vi "Dashboard Main.vi"() -> ()   [LabVIEW 2019]
uses:
  <vilib>/Rock Robotics/WPI/Camera/WPI_CameraSettings Read MJPG.ctl
  <vilib>/Rock Robotics/WPI/Camera/WPI_CameraImageSize.ctl
  Support Code/Adaptive Diagnostics/AD Status.ctl
  <vilib>/Rock Robotics/Network Tables/NT Read Number.vi
  <vilib>/Rock Robotics/Network Tables/NT Read Variant.vi
  <vilib>/Rock Robotics/Network Tables/NT Read Boolean.vi
  <vilib>/Rock Robotics/WPI/Dashboard/WPI_DashboardLogging Global.vi
  <vilib>/picture/picture.llb/Draw True-Color Pixmap.vi
  <vilib>/Rock Robotics/Network Tables/NT Read String Array.vi
  <vilib>/Rock Robotics/Network Tables/NT Write String Array.vi
  <vilib>/Rock Robotics/Network Tables/NT Write Boolean.vi
  <vilib>/Utility/miscctls.llb/LVPointTypeDef.ctl
  <vilib>/Utility/miscctls.llb/LVBoundsTypeDef.ctl
  <vilib>/FTP/NI_FTP.lvlib
  <vilib>/Rock Robotics/Network Tables/NT Write Number.vi
  <vilib>/Rock Robotics/Network Tables/NT Read String.vi
panel:
  in  "Enum":T1
  out "Camera Perf":string
  out "Right Camera Perf":cluster{"Bandwidth (Mbps)":dbl, "FPS":dbl}
  in  "Camera Settings Right":T2={"Frame Rate"=30, "Compression"=30, "Size"=1, "DB Camera Config"=FALSE} {"Frame Rate" scale=1.0..30.0; "Compression" scale=100.0..-1.0; "Size" items=["640x480", "320x240", "160x120"]}
  in  "Camera Name Right":string(combo)="No Camera Selection"
  in  "TCP":refnum<k5>
  in  "Rec Mode":enum32{"Stop", "Record", "Playback"}(radio)
  out "Robot IP":string
  in  "Dashboard Tab":T3(tab)
  out "NT 1":bool
  out "IMU 1":bool
  out "AD 1":bool
  out "Target Angle":dbl
  out "Actual Angle":dbl
  out "Target RPM":dbl
  out "Actual RPM":dbl
  in  "Camera Settings":T4={"fps"=30, "compression"=30, "Image Size"=enum."320x240", "Config Shown"=FALSE}
  out "Time Remaining":dbl
  out "Camera Image Right":T6(plugin-control)
  out "Endgame?":bool
  in  "Starting Position":bool
  in  "Remove Item":bool
  in  "Selected Item":i64
  in  "Name":string
  in  "Save":bool
  in  "Preset Auto":u16(ring) items=["3 and 3 - Left - U - Border"=1, "3 and 3 on the run- Left - U - Border"=2, "6 Ball - Center - S - Trench"=3, "6 Ball - Left - U - Border"=4, "8 Ball - Left Trench"=5, "8 Ball Right-Side"=6, "Auto test"=7, "Circles for Days"=8, "Newest"=9, "Test Code"=10, "test new"=11]
  in  "Auto Selection":u16[](array[ring]) items=["(0) 10 ft {5v 10a 0s 0f}"=1, "(0) Circle thing EXP"=2, "(0) Circle thing End"=3, "(0) Circle thing Middle"=4, "(0) Circle thing Start"=5, "(0) Circle thing {4v 20a 0s 0f}"=6, "(1) Off of hab {5v 10a 0s 5f}"=7, "0000 - REMOVE - 0000"=8, "10 feet"=9, "2056 Style Hatch Movement"=10, "Auto test 2"=11, "Auto-Builder-Test"=12, "Backup (V2) {6v, 15a, 0s. 0f}"=13, "Backup (V3) {6v, 15a, 0s. 0f}"=14, "Backup {6v, 15a, 0s. 0f}"=15, "C to shoot - Left Trench to Left Border"=16, "C to shoot - Left border"=17, "C to shoot - Trenchside border"=18, "Cargo Movement 1"=19, "Cargo Movement 2"=20, "Move to Back Trench - Front Trench"=21, "Move to Front Trench - Back Trench"=22, "Move to Front Trench for Center Port - Back Trench"=23, "Move to Front Trench for Center Port For 8 ball - Back Trench"=24, "Move to pick up 3 - Left border"=25, "Only pick up 3 - Left border"=26, "Pick up 2 - Left Trench"=27, "Pick up 2- Trenchside border"=28, "Pick up 3 - Left border"=29, "Pick up 3 - On the run border"=30, "Pick up 3 - Trench"=31, "Pick up 3 - Trench J"=32, "Pick up 3 - Trench S"=33, "Pick up 3 - Trench S + 2"=34, "Pick up 3 - Trench S + C"=35, "Pick up 3 - Trench S for 8 Ball Auto"=36, "Pick up 3 test"=37, "Shoot 3 - Center Init Line"=38, "Shoot 3 - Center Init Line Facing Left"=39, "Shoot 3 - Center Init Line Strait"=40, "Shoot 3 - Front Trench"=41, "Shoot 3 - Front and side of trench"=42, "Shoot 3 - Front and side of trench and pickup"=43, "Shoot 3 - Side of Trench"=44, "Shoot 3 and 3 - Center Init Line Facing Left"=45, "Shoot 3 and 3 - Center Init Line Facing Right"=46, "Shoot 3 and 3 on the run - Center Init Line Facing Left"=47, "Test part 1"=48, "Test part 2"=49, "Turn in place and shoot"=50, "Untitled"=51]
  in  "Re-Calibrate":bool
  out "IMU Temp":dbl
  out "Gauge":dbl(knob) scale=-10.0..10.0
  out "Picture 2":picture
  out "Mode":T7(ring)=enum."Auto Disabled"
  out "IMU Angle":dbl
  out "Network Table 2":bool
  out "IMU 2":bool
  out "Adaptive Diagnostics 2":bool
  out "Drive Base":bool
  out "Turret":bool
  out "Shooter":bool
  out "Accelerator":bool
  out "Transfer":bool
  out "Funnel":bool
  out "Intake Rotation":bool
  out "Intake Power":bool
  out "Hang":bool
  out "Clang":bool
  out "Errors":string
  out "Front Left US":bool
  out "Back Left US":bool
  out "Front Right US":bool
  out "Back Right US":bool
  out "Beam-break":bool
  out "Limellight":bool
  out "Basler":bool
  in  "AD Save Path":path
  out "Network Table 3":bool
  out "IMU 3":bool
  out "Adaptive Diagnostics 3":bool
  out "Tree":string(tree)
  # "Straight on"
  # "Jail for random constants and stuff"
  # "HW"
  # "Preset Auto Selection"
  # "Robot Health"
  # "These only run when in the programming tab"
  # "Motors show if they detect non-\nzero encoder velocity"
  # "<Side pic of robot>"
  # "US shows <10"
  # "BB shows break"
  # "LL shows coms"
  # "<Top pic of robot>"
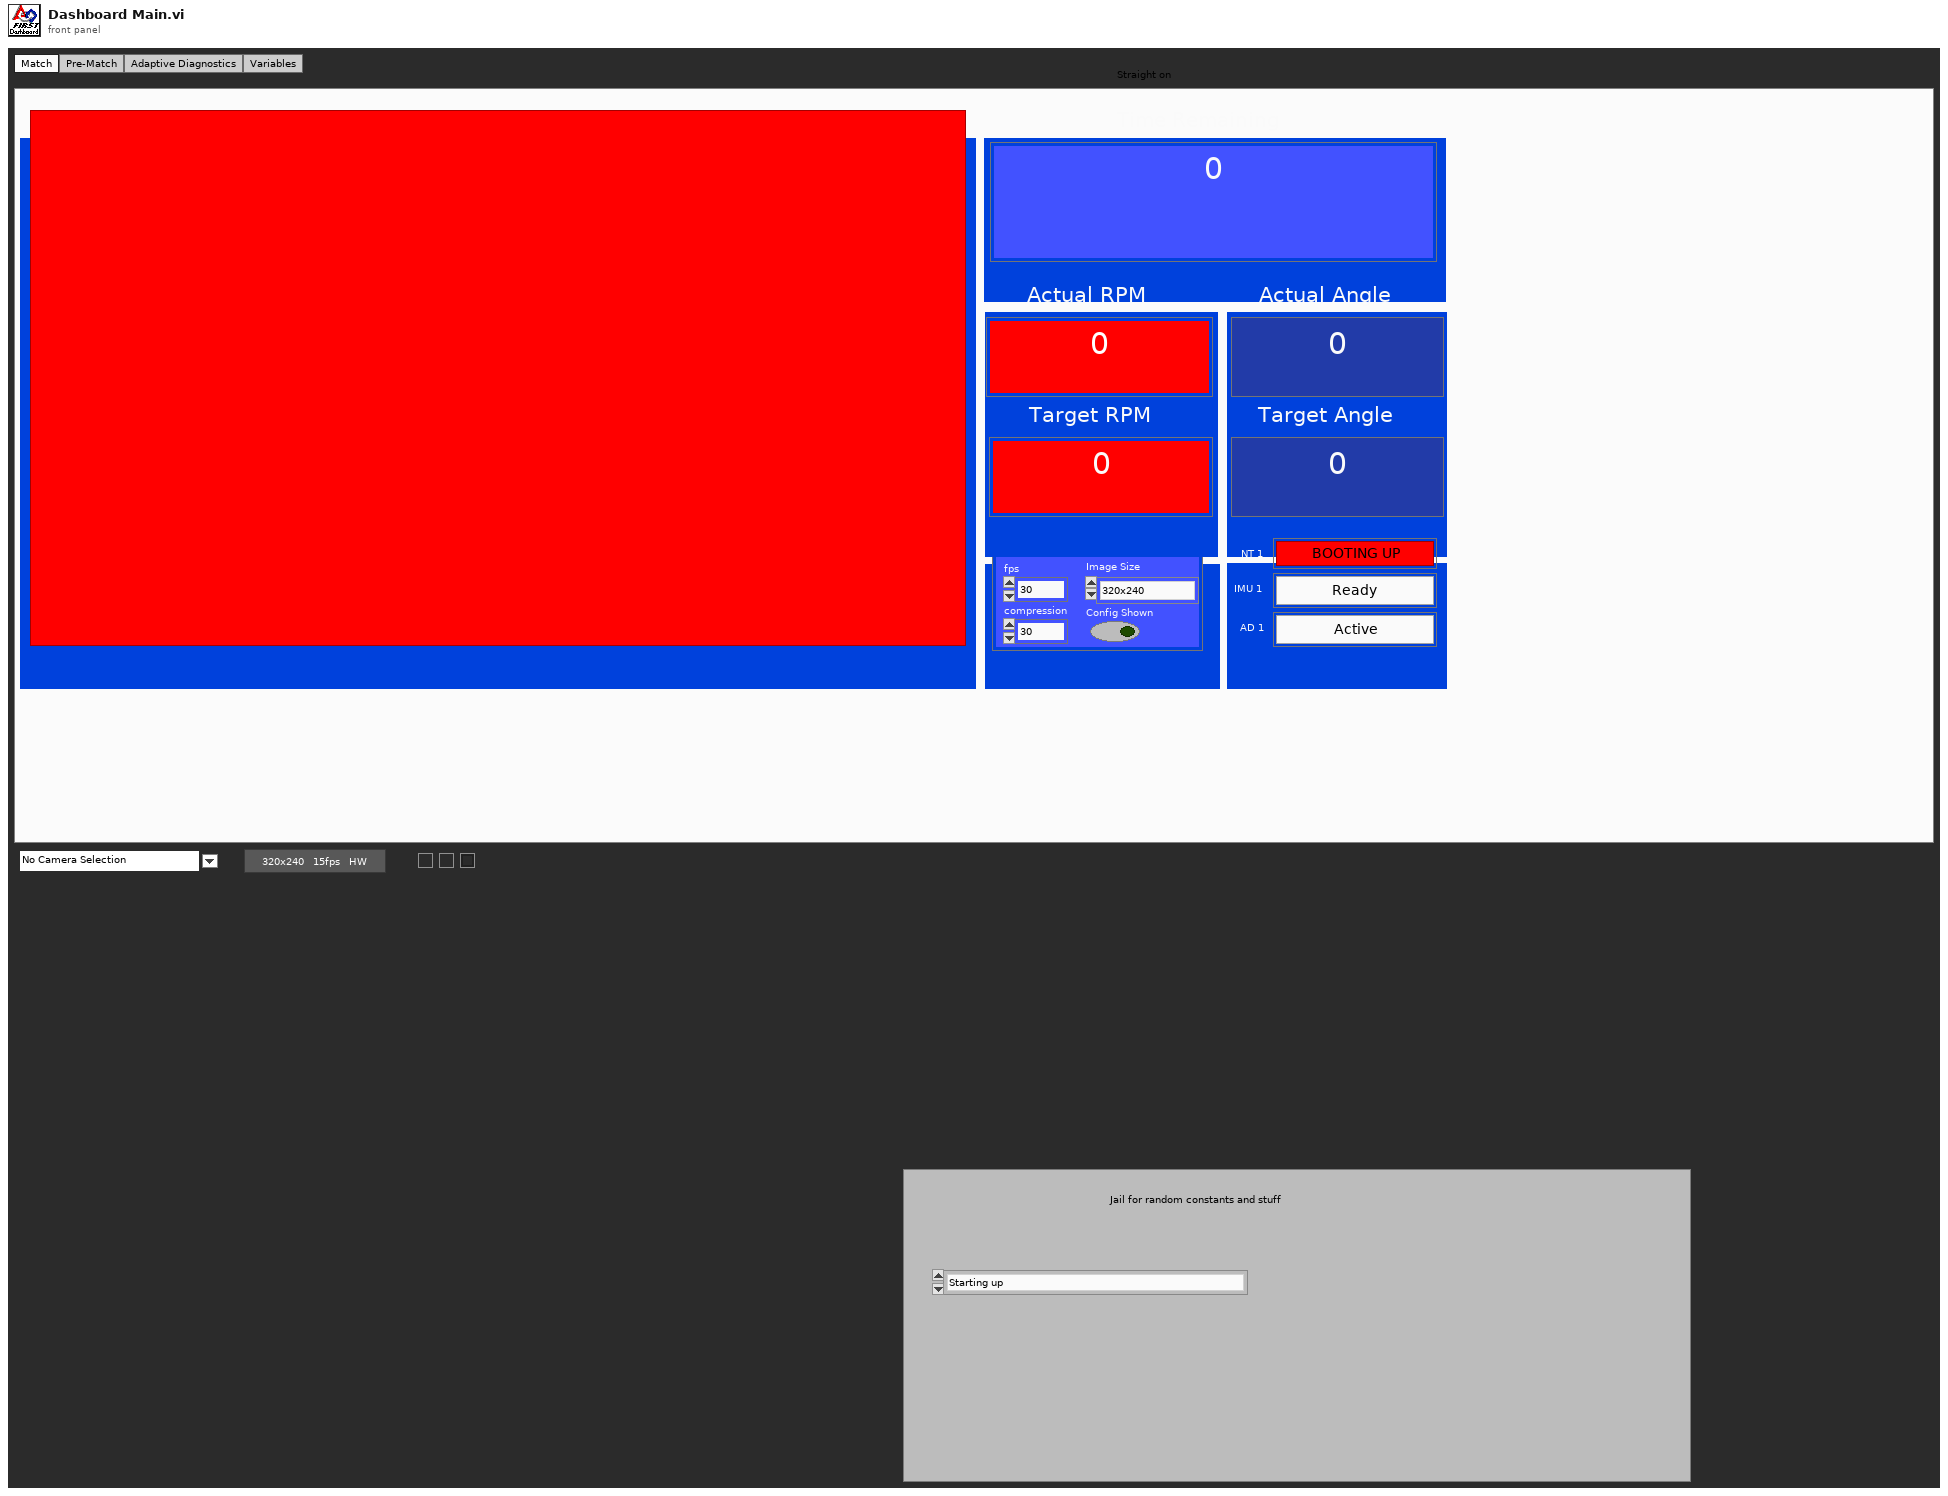
[diagram p1: front panel]
types:
  T1 = typedef "AD Status.ctl" = enum16{"Starting up", "Active", "Transfering Data", "Done"}
  T2 = cluster{"Frame Rate":i32, "Compression":i32, "Size":u16, "DB Camera Config":bool}
  T3 = enum32{"Match", "Pre-Match", "Adaptive Diagnostics", "Variables"}
  T4 = typedef "WPI_CameraSettings Read MJPG.ctl" = cluster{"fps":i32, "compression":i32, "Image Size":T5, "Config Shown":bool}
  T5 = typedef "WPI_CameraImageSize.ctl" = enum16{"640x480", "320x240", "160x120", "Custom"}
  T6 = typedef "IMAQ Image.ctl" = refnum<image>
  T7 = enum8{"Tele-Op Disabled", "Tele-Op Enabled", "Auto Disabled", "Auto Enabled", "Test Disabled", "Test Enabled", "Disconnected", "No Code", "E-Stop"}
  T8 = cluster{"Save Path":path, "Interval (s)":dbl, "Keep":i32}
  T9 = typedef "Image Type" = u32
  T10 = cluster{"IDs":cluster{"RPC field ID":u16, "Unique ID":u16}, "String":string}
  T11 = enum32{"Drive", "Camera", "Basic", "Custom", "Test", "Commands", "Checklist", "Variables"}
  T12 = cluster{"Segment Name":string, "Type":enum16{"Accel Straight", "Const Straight", "Blend", "Circle"}, "Traj Pos Points":cluster{"x":dbl, "y":dbl, "th":dbl}[], "Traj Vel Points":cluster{"V":dbl, "th":dbl}[], "Accel Index":i32, "Decel Index":i32}[]
  T13 = cluster{"Index":i32, "Pt Test Results":enum16{"Miss", "Rect Hit", "Arrow Hit"}}
  T14 = cluster{"Error Strings":string, "Disable Counts":cluster{u16, u16}, "Rail Faults":cluster{u16, u16, u16}, "Robot IP":string, "DB Mode":u8, "Event Info":cluster{"Name":string, "Type":u8, "Number":u16, "Replay":u8}}
  T15 = cluster{"Storage":cluster{"Disk Free":u64, "RAM Block":u32, "RAM free":u32}, "CPU Utilization":cluster{"CPU % ISR":sgl, "CPU % Time Crit":sgl, "CPU % Timed Str":sgl, "CPU % High":sgl, "CPU % Above":sgl, "CPU % Normal":sgl, "CPU % Low":sgl}, "CAN":cluster{"% Bus Utilization":sgl, "Bus Off Cnt":u32, "TX_FIFO Full Cnt":u32, "Receive Error Cnt":u8, "Transmit Error Cnt":u8}, "HID":cluster{"HID Outputs":u32, "Rumble Low":u16, "Rumble High":u16}[]}
  T16 = cluster{"Status bits":cluster{"Test Mode":bool, "Autonomous":bool, "Enabled":bool, "Code Start":bool, "Brownout":bool, "Reserved 2":bool, "Reserved 3":bool, "E-Stop":bool}, "Code Trace":cluster{"Disabled":bool, "TeleOp":bool, "Auto":bool, "Test":bool}, "Controller Type":enum16{"unknown", "cRIO", "roboRio"}, "Code?":enum16{"unknown", "noCode", "code"}, "Battery V":dbl}
  T17 = cluster{"Control Bits":cluster{"TestMode":bool, "Autonomous":bool, "Enabled":bool, "FMS Present":bool, bool, bool, bool, "E-Stop":bool}, "Team Station ":u8, "Countdown":sgl, "Joystick Values":cluster{"Axes":dbl[], "Buttons":bool[], "POVs":i16[]}[]}
  T18 = cluster{"Axes":dbl[], "Buttons":bool[], "POVs":i16[]}[]
  T19 = cluster{"Points":cluster{"x":dbl, "y":dbl, "th":dbl}[], "Trajectory Data":cluster{"Segment Name":string, "Type":enum16{"Accel Straight", "Const Straight", "Blend", "Circle"}, "Traj Pos Points":cluster{"x":dbl, "y":dbl, "th":dbl}[], "Traj Vel Points":cluster{"V":dbl, "th":dbl}[], "Accel Index":i32, "Decel Index":i32}[]}
  T20 = cluster{"Points":cluster{"x":dbl, "y":dbl, "th":dbl}[], "Trajectory Data":cluster{"Segment Name":string, "Type":enum16{"Accel Straight", "Const Straight", "Blend", "Circle"}, "Traj Pos Points":cluster{"x":dbl, "y":dbl, "th":dbl}[], "Traj Vel Points":cluster{"V":dbl, "th":dbl}[], "Accel Index":i32, "Decel Index":i32}[]}[]
  T21 = cluster{"Horizontal":dbl, "Vertical":dbl, "th":dbl}
  T22 = cluster{"Axes":dbl[], "Buttons":bool[], "POVs":i16[]}
  T23 = cluster{"Global Rectangle":i32[], "Contours":cluster{"Contour Type":u32, "ROI Type":u32, "Points":i32[]}[]}
  T24 = cluster{"Camera Name Right":string, string, "Saved DB Images Info":cluster{"Save Path":path, "Interval (s)":dbl, "Keep":i32}}
  T25 = cluster{"Operation":enum16{"Update", "Clear"}, "Color Box":u32}[]
  T26 = cluster{"Image Size":bool, "Image Type":bool, "Pixel Value":bool, "ROI Information":bool, "Zoom Factor":bool}
  T27 = cluster{"Shift":bool, "Ctrl":bool, "Alt":bool, "Cmd":bool, "Opt":bool}
  T28 = enum16{"open", "replace", "create", "open or create", "replace or create", "replace or create with confirmation"}
  T29 = typedef "LVBoundsTypeDef.ctl" = cluster{"Width":u32, "Height":u32}
  T30 = typedef "imagedata.ctl" = cluster{"image type":i32, "image depth":i32, "image":u8[], "mask":u8[], "colors":u32[], "Rectangle":cluster{"left":i16, "top":i16, "right":i16, "bottom":i16}}
  T31 = cluster{"Trajectory Data":cluster{"Segment Name":string, "Type":enum16{"Accel Straight", "Const Straight", "Blend", "Circle"}, "Traj Pos Points":cluster{"x":dbl, "y":dbl, "th":dbl}[], "Traj Vel Points":cluster{"V":dbl, "th":dbl}[], "Accel Index":i32, "Decel Index":i32}[], "Points":cluster{"x":dbl, "y":dbl, "th":dbl}[]}[]
  T32 = typedef "LVRectTypeDef.ctl" = cluster{"Left":i16, "Top":i16, "Right":i16, "Bottom":i16}
  T33 = typedef "LVPointTypeDef.ctl" = cluster{"Horizontal":i16, "Vertical":i16}
  T34 = enum8{"Enabled", "Disabled", "Disabled and Grayed Out"}
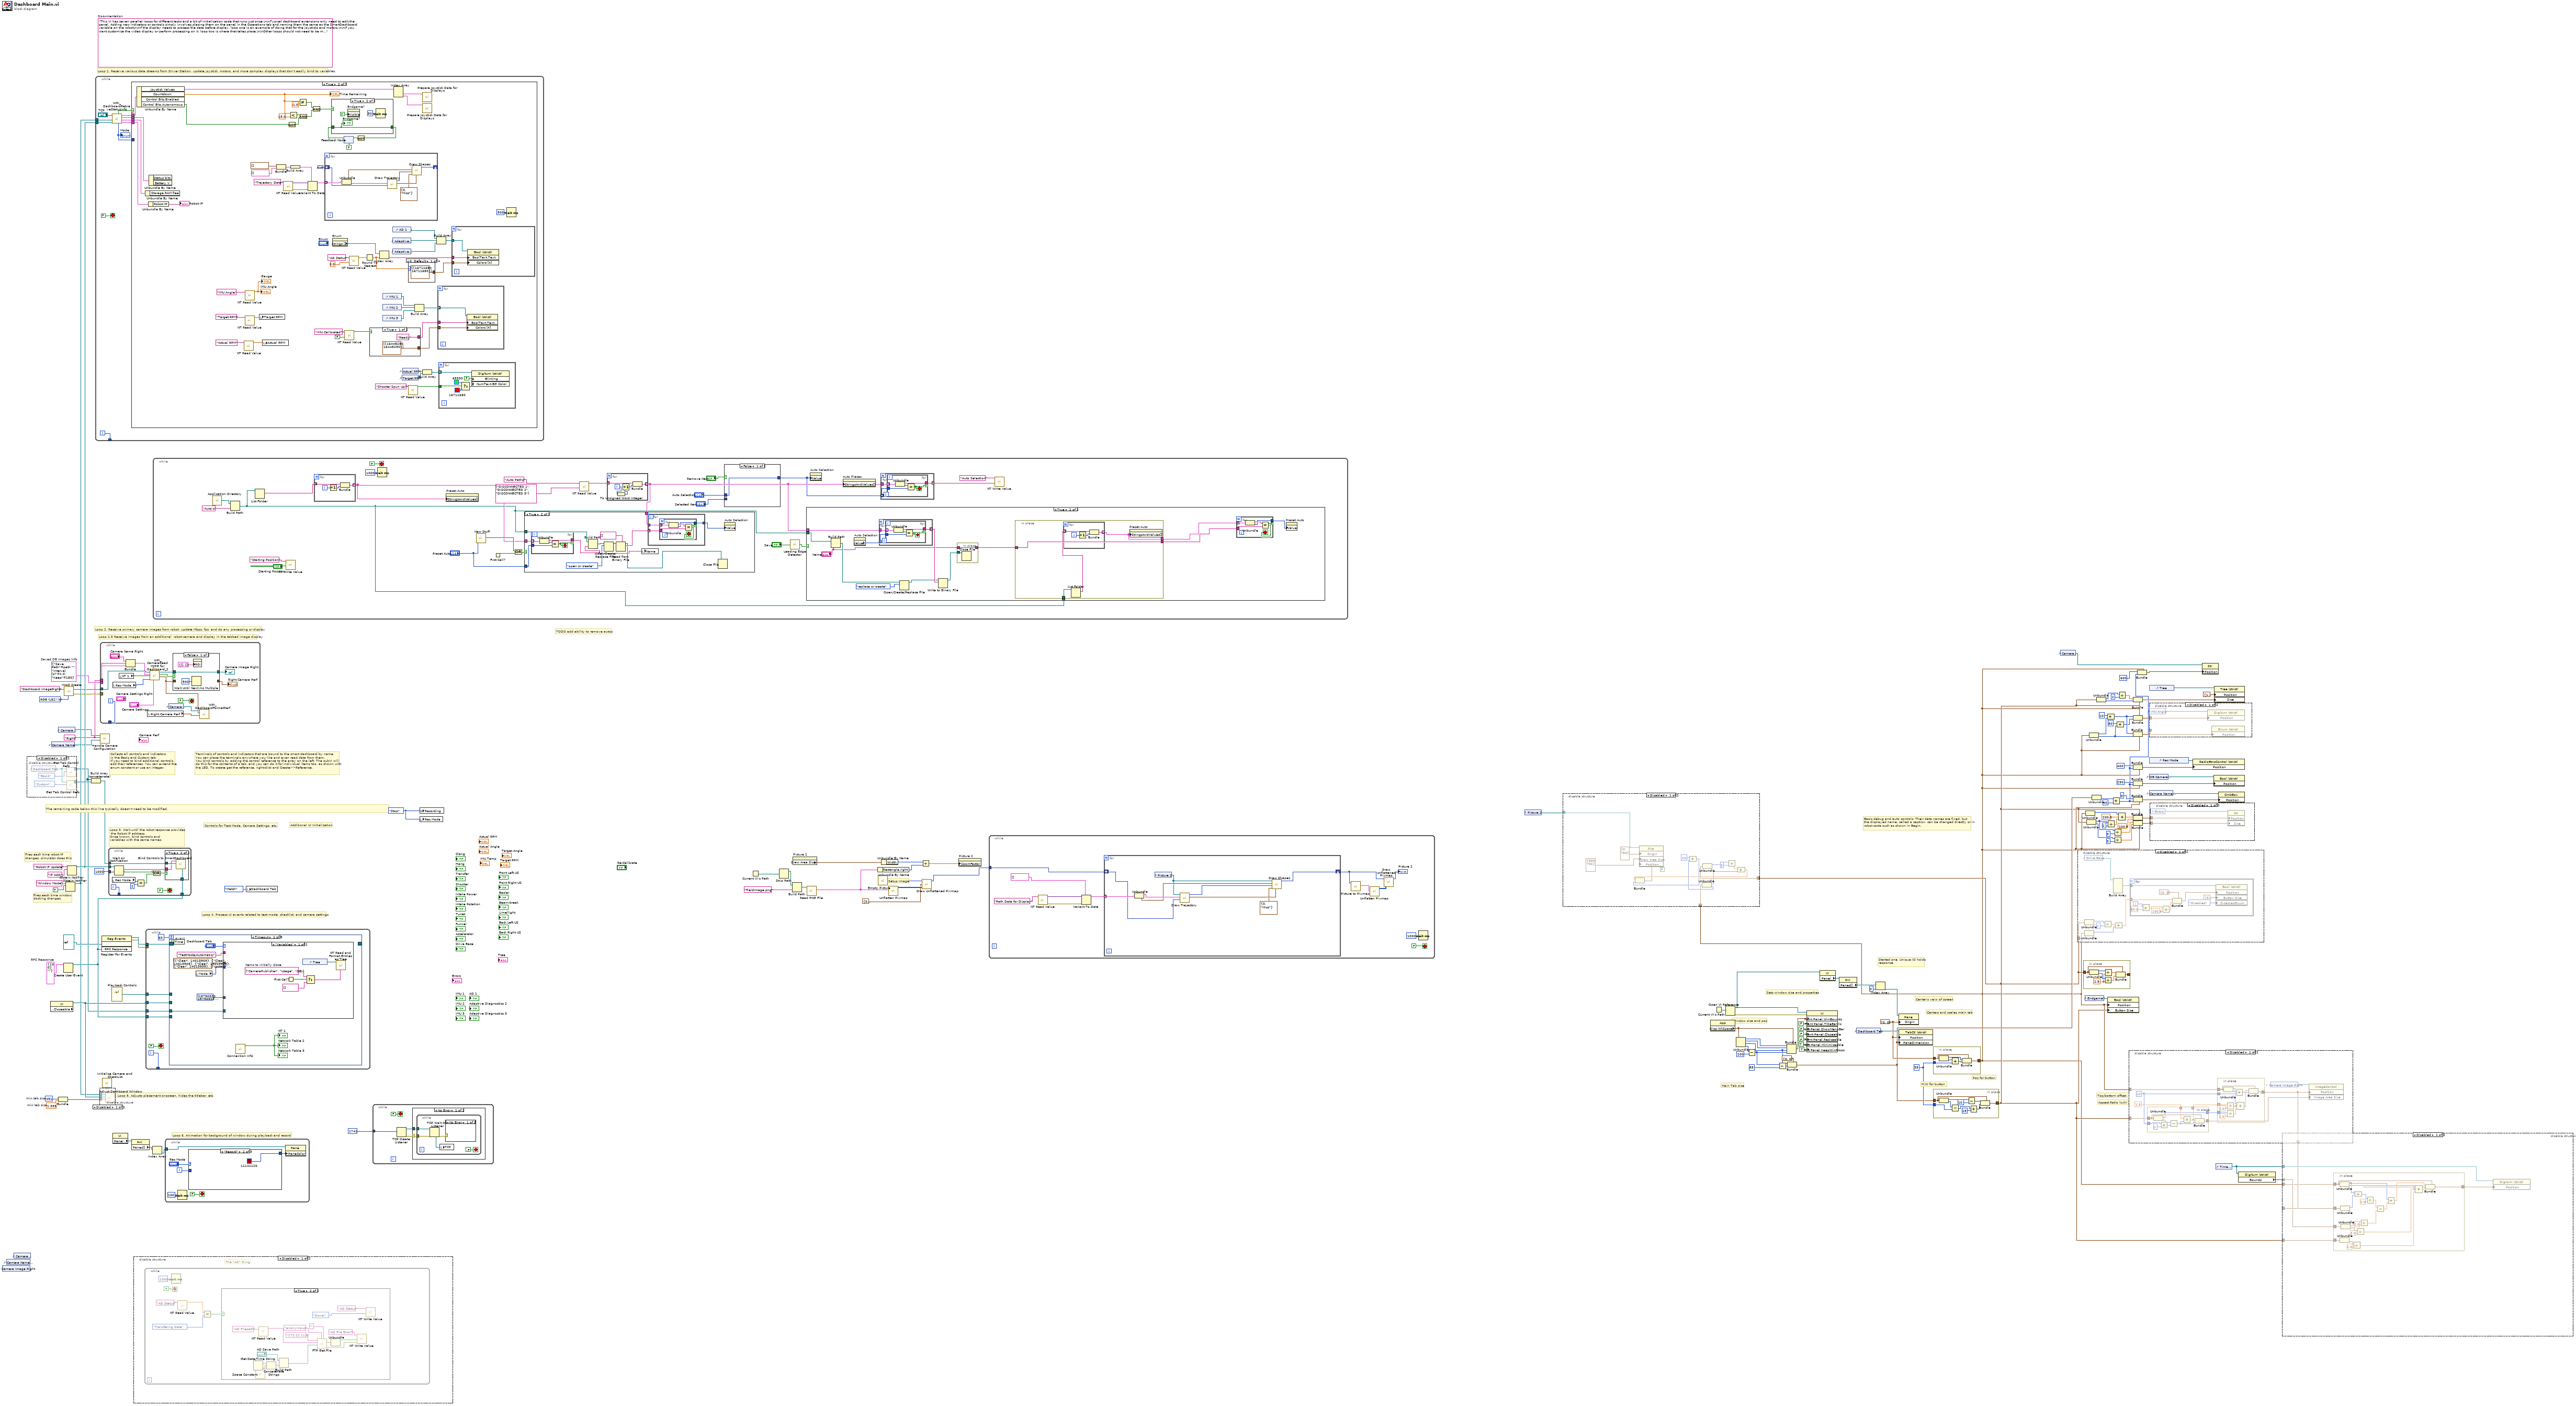
[diagram p0: block diagram]
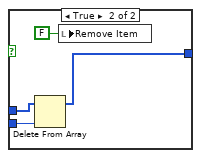
[diagram p4: hidden frame]
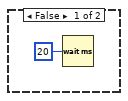
[diagram p7: hidden frame]
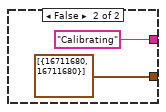
[diagram p8: hidden frame]
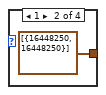
[diagram p9: hidden frame]
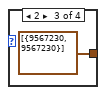
[diagram p10: hidden frame]
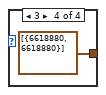
[diagram p11: hidden frame]
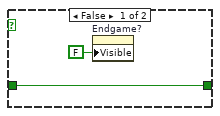
[diagram p12: hidden frame]
diagram:
  w66 = 35 ("y")
  w67 = cluster{"X":i32, "Y":i32} {"X"=0, "Y"=0}
  w95 = T8 {"Save Path"=path "", "Interval (s)"=1.0, "Keep"=180}  # Saved DB Images Info
  w94 = "Right"
  w100 = T9 4 items=["Grayscale (U8)", "Grayscale (I16)", "Grayscale (SGL)", "Complex (CSG)", "RGB (U32)", "HSL (U32)", "RGB (U64)"] ("Image Type")
  w104 = T10 {"IDs"={"RPC field ID"=0, "Unique ID"=0}, "String"=""}  # RPC Response
  w110 = 491  # min tab size
  w109 = 1.333  # min tab size
  w114 = enum32{"Stop", "Record", "Playback"}."Stop" ("Rec Mode")
  (unwired) "This VI has seven parallel loops for different tasks and a bit of initialization code that runs just once.\n\nTypical dashboard extensions only need to edit the panel. Adding new indicators or controls simply involves placing them on the panel in the Operations tab and naming them the same as the SmartDashboard variable on the robot\n\nIf the display needs to process the data before display, loop one is an example of doing that for the joysticks and motors.\n\nIf you want customize the video display or perform processing on it, loop two is where that takes place.\n\nOther loops should not need to be modified. They are pretty standard, and document the task they perform."  # Documentation
  # "TODO add ability to remove autos"
  # "Setup Image"
  # "Aspect Ratio (w/h)"
  # "Top/bottom offset"
  # "H/W for button"
  # "Pos for button"
  # "Centers and scales main tab"
  # "Center's veiw of screen"
  # "Main Tab size"
  # "Window size and pos"
  # "Sets window size and properties"
  # "Loop 2.5 Receive images from an additional  robot camera and display in the tabbed image display"
  # "Started one, Unique ID holds\nresponse"
  # "Basic debug and auto controls: Their data names are fixed, but\nthe displayed name, called a caption, can be changed directly or in\nrobot code such as shown in Begin."
  # "Controls for Test Mode, Camera Settings, etc."
  # "Additional UI Initialization"
  # "Loop 6. Animation for background of window during playback and record"
  # "Fires each time robot IP\nchanges, simulator does this"
  # "Fires each time window\ndocking changes."
  # "Collects all controls and indicators\nin the Basic and Custom tab.\nIf you need to bind additional controls,\nadd their references. You can extend the\nenum constant or use an integer."
  # "The remaining code below this line typically doesn't need to be modified."
  # "Loop 4. Process UI events related to test mode, checklist, and camera settings"
  # "Terminals of controls and indicators that are bound to the smart dashboard by name.\nYou can place the terminals anywhere you like and even read data from them.\nYou bind controls by adding the control reference to the array on the left. The subVI will\ndo this for the contents of a tab, and you can do it for individual items too, as shown with\nthe LED. To create get the reference, right-click and Create>>Reference."
  # "Loop 3. Wait until the robot response provides\n the Robot IP address.\nOnce known, bind controls and\nvariables with the same names."
  # "Loop 5. Adjusts placement onscreen, hides the titlebar, etc."
  # "Loop 1. Receive various data streams from Driver Station, update joystick, motors, and more complex displays that don't easily bind to variables."
  # "Loop 2. Receive primary camera images from robot, update Mbps, fps, and do any processing or display"
  n1 = control-ref of="Camera Image Right"() -> ()  [unwired: 1 out]
  n2 = control-ref of="Camera Name Right"() -> ()  [unwired: 1 out]
  n3 = control-ref of="Camera Settings Right"() -> ()  [unwired: 1 out]
  n4 = disable-structure shown="Disabled" {
    disable-tunnel: [w130 _] -> w112
    disable-tunnel: [w129 _] -> w102
    frame Disabled {
      n5 = control-ref of="Dashboard Tab"() -> (w131:refnum<vi>)
      n6 = call <vilib>:"Get Tab Control Refs.vi"("Page Index"=T11."Basic" ("Dashboard Tab"), "TabControl in"=w131) -> ("ControlsOnPage"=w129:refnum<vi>[])  [unwired: 9 in]
      n7 = call <vilib>:"Get Tab Control Refs.vi"("Page Index"=T11."Custom" ("Dashboard Tab"), "TabControl in"=w131) -> ("ControlsOnPage"=w130:refnum<vi>[])  [unwired: 9 in]
    }
    frame Enabled {
    }
  }
  n8 = property class="VI" props=["Front Panel.Closeable"]() -> (reference out=w113:refnum<vi>)  [unwired: 2 in, 2 out]
  n9 = control-ref of="Camera Name Right"() -> (w96:refnum<vi>)
  n10 = control-ref of="Camera Settings Right"() -> (w97:refnum<vi>)
  n11 = Bundle("min tab size"=w110, "min tab size"=w109) -> (w108:cluster{"min tab size":i32, "min tab size":dbl})  [unwired: 1 in]
  n12 = Create User Event(user event datatype=w104) -> (user event=w103:refnum<user-event>)  [unwired: 1 in, 1 out]
  n13 = call "IMAQ Create"("Image Name"="Dashboard ImageRight", "Image Type"=w100) -> ("New Image"=w99:T6, "error out"=w98:errorcluster)  [unwired: 2 in, 1 out]
  n14 = Obtain Notifier(name (unnamed)="Window Mode", notification data type=TRUE) -> (notifier out=w106:refnum<notifier>)  [unwired: 2 in, 2 out]
  n15 = Obtain Notifier(name (unnamed)="Robot IP Update", notification data type="IP Addr" ("name (unnamed)")) -> (notifier out=w107:refnum<notifier>)  [unwired: 2 in, 2 out]
  n16 = Build Array (concatenate)(w102, w112) -> (w111:refnum<vi>[])
  n17 = while {
    tunnel: [w141] -> _
    tunnel: w107 -> [w135]
    tunnel: w106 -> [w132]
    i -> [w141]
    stop <- FALSE stop-if-true
    n18 = call <vilib>:"WPI_DashboardRetrieveStatusInfo.vi"("Binding Refnum"=w135, "Window Mode Notifier"=w132, "TCP Cnx"="TCP") -> ("Power and Errors"=w136:T14, "Robot Metrics"=w139:T15, "Status Info"=w140:T16, "Control Info"=w137:T17, "Robot Mode"=w134:T7, "Process?"=w138:bool)  [unwired: 3 in]
    "Mode" <- w134
    n19 = case shown="True" w138 {
      tunnel: w140 -> [_ w205]
      tunnel: w139 -> [_ w204]
      tunnel: w137 -> [_ w203]
      tunnel: w136 -> [_ w202]
      tunnel: w134 -> [_ _]
      frame False {
        n20 = Wait (ms)(milliseconds to wait=u32 20) -> ()  [unwired: 1 out]
      }
      frame True {
        n21 = Unbundle By Name(w203) -> ("Joystick Values"=w201:T18, "Countdown"=w186:sgl, "Control Bits.Autonomous"=w197:bool)  [unwired: 1 out]
        "Time Remaining" <- w186
        n22 = Unbundle By Name(w204) -> ()  [unwired: 1 out]
        n23 = Unbundle By Name(w202) -> ("Robot IP"=→"Robot IP":string)
        n24 = Unbundle By Name(w205) -> ()  [unwired: 2 out]
        n25 = call-poly <vilib>:"NT Read Value.vi"("Name"="Actual RPM") -> ("Numeric"=w144:dbl)  [unwired: 9 in, 1 out]
        n26 = call-poly <vilib>:"NT Read Value.vi"("Name"="Target RPM") -> ("Numeric"=w147:dbl)  [unwired: 9 in, 1 out]
        n27 = call-poly <vilib>:"NT Read Value.vi"("Name"="IMU Angle") -> ("Numeric"=→"IMU Angle" →"Gauge":dbl)  [unwired: 9 in, 1 out]
        n28 = local write "Target RPM"(w147) -> ()
        n29 = local write "Actual RPM"(w144) -> ()
        n30 = Bundle("Points"=cluster{"x":dbl, "y":dbl, "th":dbl}[] [], "Trajectory Data"=T12 []) -> (w180:T19)  [unwired: 1 in]
        n31 = call-poly <vilib>:"NT Read Value.vi"("Name"="Trajectory Data") -> ("error out"=w181:errorcluster, "Variant"=w182:variant)  [unwired: 9 in]
        n32 = Not(x=w197) -> (.not. x?=w196:bool)
        n33 = Less?(x=w186, y=sgl 15.0) -> (x < y?=w195:bool)
        n34 = Build Array(w180) -> (w179:T20)
        n35 = Not Equal?(x=w186, y=sgl -1.0) -> (x != y?=w188:bool)
        n36 = And(x=w195, y=w196) -> (x .and. y?=w187:bool)
        n37 = Variant To Data(error in=w181, type=w179, Variant=w182) -> (data=w178:T20)  [unwired: 1 out]
        n38 = And(x=w188, y=w187) -> (x .and. y?=w185:bool)
        n39 = for {
          tunnel: w178 -> [w227] mode=indexing
          shift-right: [w231] -> _
          shift-left: picture data[5B] ("new picture out") -> [w226]
          n40 = Unbundle(w227) -> ("Points"=w229:cluster{"x":dbl, "y":dbl, "th":dbl}[], "Trajectory Data"=w228:T12)
          n41 = call "Draw Trajectory.vi"("new picture in"=w226, "Trajectory Data"=w228) -> ("Output Point"=w233:T21, "new picture"=w232:picture)  [unwired: 8 in]
          n42 = call "Draw Shapes.vi"("Output Point"=w233, "Results"=T13 {"Index"=0, "Pt Test Results"=enum."Miss"}, "new picture in"=w232, "Points"=w229) -> ("new picture out"=w231:picture)  [unwired: 7 in]
        }
        n43 = property on="Enum" class="Enum (strict)"() -> ("Strings []"=w169:string[])  [unwired: 2 in, 2 out]
        n44 = feedback #1(FALSE ("Endgame?")) -> (w191:bool)
        n45 = call-poly <vilib>:"NT Read Value.vi"("Default Value"=FALSE, "Name"="IMU Calibrated?") -> ("Boolean"=w164:bool)  [unwired: 8 in, 1 out]
        n46 = call-poly <vilib>:"NT Read Value.vi"("Default Value"=0.0, "Name"="AD Status") -> ("Numeric"=w172:dbl)  [unwired: 8 in, 1 out]
        n47 = Not(x=w191) -> (.not. x?=w190:bool)
        n48 = case shown="True" w185 {
          tunnel: [w235 w238] -> w192
          tunnel: w190 -> [w235 w238]
          frame False {
            n49 = property on="Endgame?" class="Bool (strict)"("Visible"=FALSE) -> ()  [unwired: 2 in, 2 out]
          }
          frame True {
            n50 = property on="Endgame?" class="Bool (strict)"("Visible"=TRUE) -> ()  [unwired: 2 in, 2 out]
            n51 = Wait (ms)(milliseconds to wait=u32 50) -> ()  [unwired: 1 out]
            "Endgame?" <- w238
          }
        }
        n52 = feedback-in #1(w192) -> ()
        n53 = Round To Nearest(number=w172) -> (nearest integer value=w168:dbl)
        n54 = case shown="True" w164 {
          tunnel: ["Ready" ("Name") "Calibrating" ("Name")] -> w163
          tunnel: [cluster{u32, u32}[] [{16448250, 16448250}] ("Colors [4]") cluster{u32, u32}[] [{16711680, 16711680}] ("Colors [4]")] -> w162
          frame True {
          }
          frame False {
          }
        }
        n55 = Index Array(array=w169, index=w168) -> (element=w170:string)
        n56 = control-ref of="IMU 1"() -> (w157:refnum<vi>)
        n57 = control-ref of="IMU 2"() -> (w158:refnum<vi>)
        n58 = control-ref of="IMU 3"() -> (w156:refnum<vi>)
        n59 = control-ref of="AD 1"() -> (w155:refnum<vi>)
        n60 = control-ref of="Adaptive Diagnostics 2"() -> (w154:refnum<vi>)
        n61 = control-ref of="Adaptive Diagnostics 3"() -> (w153:refnum<vi>)
        n62 = Index Array(array=w201) -> (element #1=w200:T22, element #2=w199:T22)  [unwired: 2 in]
        n63 = control-ref of="Target RPM"() -> (w150:refnum<vi>)
        n64 = control-ref of="Actual RPM"() -> (w151:refnum<vi>)
        n65 = case shown="0, Default" w168 {
          tunnel: [cluster{u32, u32}[] [{16711680, 16711680}] ("Colors [4]") cluster{u32, u32}[] [{16448250, 16448250}] ("Colors [4]") cluster{u32, u32}[] [{9567230, 9567230}] ("Colors [4]") cluster{u32, u32}[] [{6618880, 6618880}] ("Colors [4]")] -> w167
          frame 0, Default {
          }
          frame 1 {
          }
          frame 2 {
          }
          frame 3 {
          }
        }
        n66 = call-poly <vilib>:"NT Read Value.vi"("Name"="Shooter Spun Up?") -> ("Boolean"=w148:bool)  [unwired: 9 in, 1 out]
        n67 = Build Array(w157, w158, w156) -> (w165:refnum<vi>[])
        n68 = call "Prepare Joystick Data for Displays.vi"("Joystick Values"=w199) -> ()  [unwired: 8 in, 3 out]
        n69 = call "Prepare Joystick Data for Displays.vi"("Joystick Values"=w200) -> ()  [unwired: 8 in, 3 out]
        n70 = Build Array(w151, w150) -> (w152:refnum<vi>[])
        n71 = Build Array(w155, w154, w153) -> (w171:refnum<vi>[])
        n72 = for {
          tunnel: w165 -> [w218] mode=indexing
          tunnel: w163 -> [w217]
          tunnel: w162 -> [w216]
          n73 = property class="Bool (strict)"(reference=w218, "BoolText.Text"=w217, "Colors [4]"=w216) -> ()  [unwired: 1 in, 2 out]
        }
        n74 = for {
          tunnel: w152 -> [w211] mode=indexing
          tunnel: w148 -> [w210]
          n75 = Select(t=u32 65330 ("Numeric Text.Colors:BG Color"), s=w210, f=u32 16711680 ("Numeric Text.Colors:BG Color")) -> (s? t:f=w206:u32)
          n76 = property class="DigNum (strict)"(reference=w211, "Blinking"=FALSE, "NumText.BG Color"=w206) -> ()  [unwired: 1 in, 2 out]
        }
        n77 = for {
          tunnel: w171 -> [w225] mode=indexing
          tunnel: w170 -> [w224]
          tunnel: w167 -> [w223]
          n78 = property class="Bool (strict)"(reference=w225, "BoolText.Text"=w224, "Colors [4]"=w223) -> ()  [unwired: 1 in, 2 out]
        }
        n79 = Wait (ms)(milliseconds to wait=u32 500) -> ()  [unwired: 1 out]
      }
    }
  }
  n80 = disable-structure shown="Disabled" {
    disable-tunnel: w113 -> [w241 _]
    disable-tunnel: w108 -> [w240 _]
    disable-tunnel: w106 -> [w239 _]
    frame Disabled {
      n81 = call "Adjust Dashboard Window.vi"("Size Constraints"=w240, "VI"=w241, "WIn Mode"=w239) -> ()  [unwired: 9 in]
    }
    frame Enabled {
    }
  }
  n82 = call "Handle Camera Configuration.vi"("CameraNameRef"=w96, "Display Name"=w94, "ClusterRef"=w97) -> ()  [unwired: 9 in]
  n83 = while {
    tunnel: w99 -> [w258]
    tunnel: w98 -> [_]
    tunnel: [w254] -> _
    tunnel: w95 -> [w251]
    tunnel: w94 -> [w248]
    i -> [w254]
    stop <- FALSE stop-if-true
    n84 = local read "Rec Mode"() -> (w257:enum32{"Stop", "Record", "Playback"})
    n85 = local read "NT 1"() -> (w242:bool)
    n86 = Bundle("Camera Name Right"="Camera Name Right", w248, "Saved DB Images Info"=w251) -> (w250:T24)  [unwired: 1 in]
    n87 = local read "Right Camera Perf"() -> (w245:cluster{"Bandwidth (Mbps)":dbl, "FPS":dbl})
    n88 = call <vilib>:"WPI_CameraRead MJPG for Dashboard_2.vi"("Camera Settings"="Camera Settings", "Rec Mode"=w257, "NT Connection"=w242, "Capture Info"=w250, "Image in"=w258) -> ("perf info"=w244:cluster{"Bandwidth (Mbps)":dbl, "fps":dbl}, "Active"=w253:bool, "Image\\ out"=w256:T6)  [unwired: 4 in]
    n89 = control-ref of="Camera Perf"() -> (w246:refnum<vi>)
    n90 = case shown="False" w253 {
      tunnel: w256 -> [w260 w263]
      tunnel: [w260 w263] -> w252
      tunnel: [_ w262] -> w247
      tunnel: w244 -> [_ w262]
      frame False {
        n91 = Wait Until Next ms Multiple(millisecond multiple=u32 500) -> ()  [unwired: 1 out]
        n92 = property on="Camera Image Right" class="ImageControl"("ROI"=T23 {"Global Rectangle"=[], "Contours"=[]}) -> ()  [unwired: 2 in, 2 out]
      }
      frame True {
      }
    }
    "Camera Image Right" <- w252
    "Right Camera Perf" <- w247
    n93 = call <vilib>:"WPI_DashboardFormatPerf.vi"("Right Camera Perf"=w245, "Performance"=w244, "String in"=w246) -> ()  [unwired: 9 in]
  }
  n94 = register-events(refnum<vi> refnum, w103) -> (reference out=w118:refnum<event-registration>, error out=w117:errorcluster)  [unwired: 2 in]
  n95 = call "Initialize Camera and CheckList.vi"() -> ()  [unwired: 12 in]
  n96 = while {
    tunnel: w111 -> [w275]
    tunnel: w107 -> [w273]
    tunnel: [w271] -> _
    tunnel: u32 1000 ("milliseconds to wait") -> [w270]
    tunnel: w103 -> [w264]
    i -> [w271]
    stop <- FALSE stop-if-true
    n97 = local read "Rec Mode"() -> (w266:enum32{"Stop", "Record", "Playback"})
    n98 = Wait on Notification(notifier=w273, timeout in ms (-1)=w270) -> (notification=w272:string, timed out?=w268:bool)  [unwired: 2 in, 2 out]
    n99 = Equal?(x=w266, y=u16 2 ("Rec Mode")) -> (x = y?=w267:bool)
    n100 = Compound Arithmetic op=OR(invert w268, w267) -> (w269:bool)
    n101 = case shown="True" w269 {
      tunnel: w275 -> [_ w278]
      tunnel: w272 -> [_ w277]
      tunnel: w264 -> [_ w276]
      frame False {
      }
      frame True {
        n102 = call <vilib>:"Bind Controls to SmartDashboard.vi"("RPC ref"=w276, "Bound Control Refs"=w278, "Server IP Address"=w277) -> ()  [unwired: 9 in]
      }
    }
  }
  n103 = vi-ref "Playback Controls.vi"() -> (w119:refnum<vi>)
  n104 = property class="VI"() -> ("Panel"=w121:refnum<vi>)  [unwired: 2 in, 2 out]
  n105 = property class="Pnl"(reference=w121) -> ("Panes[]"=w122:refnum<vi>[])  [unwired: 1 in, 2 out]
  n106 = disable-structure shown="Disabled" {
    frame Disabled {
      # "The \"AD\" thing"
      n107 = while {
        stop <- FALSE stop-if-true
        n108 = Wait (ms)(milliseconds to wait=u32 1000) -> ()  [unwired: 1 out]
        n109 = call-poly <vilib>:"NT Read Value.vi"("Name"="AD Status") -> ("Numeric"=w281:dbl)  [unwired: 9 in, 1 out]
        n110 = Equal?(x=w281, y=AD_Status."Transfering Data") -> (x = y?=w279:bool)
        n111 = case shown="True" w279 {
          frame False {
          }
          frame True {
            n112 = Get Date/Time String() -> (date string=w287:string, time string=w286:string)  [unwired: 3 in]
            n113 = call <vilib>:"Space Constant.vi"() -> ("String"=w288:string)
            n114 = call-poly <vilib>:"NT Read Value.vi"("Name"="AD Filepath") -> ("String"=w293:string)  [unwired: 9 in, 1 out]
            n115 = Concatenate Strings(w287, w288, w286) -> (w289:string)
            n116 = Build Path(base path="AD Save Path", name or relative path=w289) -> (appended path=w285:path)
            n117 = call <vilib>:"FTP Get File.vi"("password"="", "user"="anonymous", "local path"=w285, "remote path"=w293, "host"="172.22.11.2" ("address")) -> ("error out"=w301:errorcluster, "file error"=w299:errorcluster)  [unwired: 5 in]
            n118 = Unbundle(w299) -> ("status"=w300:bool)  [unwired: 2 out]
            n119 = call-poly <vilib>:"NT Write Value.vi"("error in"=w301, "Boolean"=w300, "Name"="AD File Error?") -> ()  [unwired: 8 in, 1 out]
            n120 = call-poly <vilib>:"NT Write Value.vi"("Numeric"=AD_Status."Done", "Name"="AD Status") -> ()  [unwired: 9 in, 1 out]
          }
        }
      }
    }
    frame Enabled {
    }
  }
  n121 = while {
    tunnel: [w307] -> _
    tunnel: w119 -> [w306]
    tunnel: w118 -> [w305]
    tunnel: w117 -> [_]
    tunnel: w113 -> [w304]
    tunnel: w103 -> [w303]
    tunnel: w102 -> [w302]
    i -> [w307]
    stop <- FALSE stop-if-true
    n122 = event shown="[0] Timeout" {
      selector: w305 -> [_ _ _ _ _]
      dyn-events: [_ w328 _ _ _] -> _
      timeout: u32 60 ("milliseconds to wait") -> [_ _ _ _ _]
      tunnel: w306 -> [_ w330 _ w346 _]
      tunnel: w304 -> [_ w326 _ _ _]
      tunnel: w303 -> [_ w324 _ _ _]
      tunnel: w302 -> [w311 _ _ _ _]
      event Timeout {
        n123 = event-data() -> ()  [unwired: 1 in, 1 out]
        n124 = local read "Mode"() -> (w314:T7)
        n125 = case shown="\"Variables\"" "Dashboard Tab" {
          tunnel: "TestMode/Automatic/" ("Name Pattern") -> [_ _]
          tunnel: T25 [{"Operation"=enum."Clear", "Color Box"=14013909}, {"Operation"=enum."Clear", "Color Box"=14013909}, {"Operation"=enum."Clear", "Color Box"=14013909}, {"Operation"=enum."Clear", "Color Box"=14013909}, {"Operation"=enum."Update", "Color Box"=14013909}, {"Operation"=enum."Update", "Color Box"=16777215}, {"Operation"=enum."Clear", "Color Box"=14013909}, {"Operation"=enum."Clear", "Color Box"=14013909}, {"Operation"=enum."Clear", "Color Box"=14013909}] -> [_ _]
          tunnel: w314 -> [_ _]
          tunnel: u32[] [15790320, 15790320, 15790320, 15790320, 16777215, 16777215, 15790320, 15790320, 15790320] -> [_ _]
          tunnel: w311 -> [_ _]
          frame "Variables" {
            w319 = string[] ["CameraPublisher", "Usage", "DB"]  # Items to initially close
            n126 = First Call?() -> (First Call?: T/F=w320:bool)
            n127 = control-ref of="Tree"() -> (w321:refnum<vi>)
            n128 = Select(t=w319, s=w320, f=string[] []) -> (s? t:f=w317:string[])
            n129 = call <vilib>:"NT Read and Format Entries as Tree.vi"("Tags to  Close"=w317, "Tree Refnum"=w321) -> ()  [unwired: 8 in, 2 out]
          }
          frame "Match", Default {
          }
        }
        n130 = call <vilib>:"Connextion Info.vi"() -> ("Connected"=→"NT 1" →"Network Table 2" →"Network Table 3":bool)  [unwired: 10 in, 1 out]
      }
      event "Rec Mode": Value Change {
        # "Update globals for recording mode and path to read log from.\nClear when logging and let NetworkTables set path for vision to\nuse."
        n131 = event-data() -> ("NewVal"=w331:enum32{"Stop", "Record", "Playback"})  [unwired: 1 in]
        n132 = global write "WPI_DashboardLogging Global.vi" "Logging Filename"(path "") -> ()
        n133 = global write "WPI_DashboardLogging Global.vi" "Recording"(w331) -> ()
        n134 = case shown="\"Playback\"" w331 {
          tunnel: w330 -> [_ w333 w342]
          tunnel: [_ _ w341] -> w328
          tunnel: [_ _ w340] -> _
          tunnel: w326 -> [_ _ w338]
          tunnel: cluster{i32, i32} {-250, 170} -> [_ _ w337]
          tunnel: [_ _ T26 {"Image Size"=TRUE, "Image Type"=TRUE, "Pixel Value"=TRUE, "ROI Information"=TRUE, "Zoom Factor"=FALSE} ("Image Information Shown:All Elements")] -> w322
          tunnel: [_ _ TRUE ("Zoom Factor")] -> w323
          tunnel: w324 -> [_ _ w334]
          frame Default {
          }
          frame "Stop", "Record" {
            # "Place Window too"
            n135 = invoke class="VI" method="FP.Close"(reference=w333) -> (reference out=w332:refnum<vi>)  [unwired: 2 in, 2 out]
            n136 = invoke class="VI" method="Abort VI"(reference=w332) -> ()  [unwired: 2 in, 3 out]
          }
          frame "Playback" {
            n137 = call "Open Playback Panel.vi"("Offset"=w337, "DB VI Ref"=w338, "Playback in"=w342) -> ("Playback out"=w339:refnum<vi>)  [unwired: 8 in]
            n138 = register-events(w339, w334) -> (reference out=w341:refnum<event-registration>, error out=w340:errorcluster)  [unwired: 2 in]
          }
        }
        n139 = property on="Camera Image Right" class="ImageControl"("Image Information Shown"=w322, "Image Information Visible"=w323) -> ()  [unwired: 2 in, 2 out]
        n140 = call <vilib>:"WPI_DashboardNT Log FieldName Cache.vi"("Operation"=enum16{"Lookup/Add", "Index", "Clear"}."Clear") -> ()  [unwired: 8 in, 3 out]
      }
      event Panel Close {
        w343 = enum32{"Stop", "Record", "Playback"}."Stop" ("Rec Mode")
        # "Playback window has been closed, abort"
        n141 = event-data() -> ()  [unwired: 1 in, 4 out]
        n142 = local write "Rec Mode"(w343) -> ()
        n143 = global write "WPI_DashboardLogging Global.vi" "Recording"(w343) -> ()
      }
      event Panel Close {
        # "Abort playback window and ourself"
        n144 = event-data() -> ()  [unwired: 1 in, 4 out]
        n145 = invoke class="VI" method="FP.Close"(reference=w346) -> (reference out=w345:refnum<vi>)  [unwired: 2 in, 2 out]
        n146 = invoke class="VI" method="Abort VI"(reference=w345) -> (error out=w344:errorcluster)  [unwired: 2 in, 2 out]
        n147 = invoke class="VI" method="Abort VI"(error in=w344) -> ()  [unwired: 2 in, 3 out]
      }
      event "Tree": Double Click {
        n148 = event-data() -> ("PlatMods"=w352:T27, "Tag"=w349:string)  [unwired: 1 in]
        n149 = Unbundle(w352) -> ("Shift"=w351:bool)  [unwired: 4 out]
        n150 = String Subset(string=w349, length (rest)=1 ("length (rest)")) -> (substring=w348:string)  [unwired: 1 in]
        n151 = Not(x=w351) -> (.not. x?=w350:bool)
        n152 = case shown="\"/\"" w348 {
          tunnel: w349 -> [_ w354]
          tunnel: w350 -> [_ w353]
          frame Default {
          }
          frame "/" {
            n153 = call <vilib>:"NT Update Persistence.vi"("Persistence"=w353, "Name"=w354) -> ()  [unwired: 9 in, 1 out]
          }
        }
      }
    }
  }
  n154 = Index Array(array=w122) -> (element=w120:refnum<vi>)  [unwired: 1 in]
  n155 = while {
    stop <- FALSE stop-if-true
    n156 = call <vilib>:"Application Directory.vi"() -> ("Application Directory"=w359:path)
    n157 = Build Path(base path=w359, name or relative path="Auto's") -> (appended path=w357:path)
    n158 = List Folder(path=w357) -> (filenames=w374:string[])  [unwired: 3 in, 3 out]
    n159 = call-poly <vilib>:"NT Write Value.vi"("Boolean"="Starting Position", "Name"="Starting Position") -> ()  [unwired: 9 in, 1 out]
    n160 = for {
      tunnel: w374 -> [w456] mode=indexing
      tunnel: [w455] -> w368 mode=indexing
      i -> [w458]
      n161 = Increment(x=w458) -> (x+1=w457:i32)
      n162 = Bundle(w456, w457) -> (w455:cluster{string, i32})  [unwired: 1 in]
    }
    n163 = Wait (ms)(milliseconds to wait=u32 1000) -> ()  [unwired: 1 out]
    n164 = property on="Preset Auto" class="Ring (strict)"("StringsAndValues[]"=w368) -> ()  [unwired: 2 in, 2 out]
    n165 = call "New Stuff.vi"("Variant 14"="Preset Auto") -> ("x != y?"=w371:bool)  [unwired: 26 in]
    n166 = First Call?() -> (First Call?: T/F=w372:bool)
    n167 = Or(x=w371, y=w372) -> (x .or. y?=w373:bool)
    n168 = call-poly <vilib>:"NT Read Value.vi"("Default Value"=string[] ["DISCONNECTED 1", "DISCONNECTED 2", "DISCONNECTED 3"], "Name"="Auto Paths") -> ("String Array"=w379:string[])  [unwired: 8 in, 1 out]
    n169 = for {
      tunnel: w379 -> [w462] mode=indexing
      tunnel: [w461] -> w365 mode=indexing
      i -> [w460]
      n170 = To Unsigned Word Integer(number=w460) -> (unsigned 16bit integer=w459:u16)
      n171 = Increment(x=w459) -> (x+1=w463:u16)
      n172 = Bundle("String"=w462, w463) -> (w461:cluster{"String":string, u16})  [unwired: 1 in]
    }
    n173 = case shown="True" w373 {
      tunnel: w357 -> [_ w441]
      tunnel: w365 -> [_ w435]
      tunnel: w368 -> [_ w432]
      tunnel: "Preset Auto" -> [_ w431]
      frame False {
      }
      frame True {
        n174 = for {
          tunnel: w432 -> [w446] mode=indexing
          tunnel: w431 -> [w444]
          tunnel: [w445] -> w430 if=w442
          stop <- w442 stop-if-true
          n175 = Unbundle(w446) -> (w445:string, w443:i32)
          n176 = Equal?(x=w443, y=w444) -> (x = y?=w442:bool)
        }
        n177 = Build Path(base path=w441, name or relative path=w430) -> (appended path=w440:path)
        n178 = Open/Create/Replace File(file path (use dialog)=w440, operation (0:open)=T28."open or create") -> (refnum out=w438:refnum<file>)  [unwired: 4 in, 2 out]
        n179 = Read from Binary File(5:string[] [], 11:w438) -> (2:w436:string[], 3:w433:refnum<file>)  [unwired: 4 in, 2 out]
        n180 = local write "Name"(w430) -> ()
        n181 = for {
          tunnel: w436 -> [w448] mode=indexing
          tunnel: w435 -> [w449]
          tunnel: [w447] -> w434 mode=indexing
          n182 = for {
            tunnel: w449 -> [w454] mode=indexing
            tunnel: w448 -> [w452]
            tunnel: [w451] -> w447 if=w450
            stop <- w450 stop-if-true
            n183 = Unbundle(w454) -> ("String"=w453:string, w451:u16)
            n184 = Equal?(x=w453, y=w452) -> (x = y?=w450:bool)
          }
        }
        n185 = Close File(refnum=w433) -> ()  [unwired: 1 in, 2 out]
        n186 = property on="Auto Selection" class="Arr (strict)"("Value"=w434) -> ()  [unwired: 2 in, 2 out]
      }
    }
    n187 = case shown="False" "Remove Item" {
      tunnel: "Selected Item" -> [_ w384]
      tunnel: "Auto Selection" -> [w380 w383]
      tunnel: [w380 w382] -> w360
      frame False {
      }
      frame True {
        n188 = Delete From Array(array=w383, index=w384) -> (array with subset deleted=w382:u16[])  [unwired: 1 in, 1 out]
        n189 = local write "Remove Item"(FALSE ("Remove Item")) -> ()
      }
    }
    n190 = call "Leading Edge Detector.vi"("Boolean"="Save") -> ("Out"=w370:bool)
    n191 = case shown="True" w370 {
      tunnel: w365 -> [_ w406]
      tunnel: w357 -> [_ w402]
      tunnel: w357 -> [_ w393]
      frame False {
      }
      frame True {
        n192 = Build Path(base path=w402, name or relative path="Name") -> (appended path=w401:path)
        n193 = property on="Auto Selection" class="Arr (strict)"() -> ("Value"=w405:u16[])  [unwired: 2 in, 2 out]
        n194 = for {
          tunnel: w406 -> [w424]
          tunnel: w405 -> [w423] mode=indexing
          tunnel: [w422] -> w404 mode=indexing
          n195 = for {
            tunnel: w424 -> [w429] mode=indexing
            tunnel: w423 -> [w427]
            tunnel: [w428] -> w422 if=w425
            stop <- w425 stop-if-true
            n196 = Unbundle(w429) -> ("String"=w428:string, w426:u16)
            n197 = Equal?(x=w426, y=w427) -> (x = y?=w425:bool)
          }
        }
        n198 = Open/Create/Replace File(file path (use dialog)=w401, operation (0:open)=T28."replace or create") -> (refnum out=w400:refnum<file>)  [unwired: 4 in, 2 out]
        n199 = Write to Binary File(file (use dialog)=w400, data=w404) -> (refnum out=w399:refnum<file>)  [unwired: 4 in, 2 out]
        n200 = in-place {
          in-place-border: w399 -> [w416]
          in-place-border: "Name" -> [w415]
          in-place-border: [w415] -> w395
          n201 = Close File(refnum=w416) -> ()  [unwired: 1 in, 2 out]
        }
        n202 = in-place {
          in-place-border: [w410] -> w396
          in-place-border: w395 -> [w410]
          in-place-border: [w408] -> w394
          in-place-border: w393 -> [w407]
          n203 = List Folder(path=w407) -> (filenames=w409:string[])  [unwired: 3 in, 3 out]
          n204 = for {
            tunnel: w409 -> [w412] mode=indexing
            tunnel: [w411] -> w408 mode=indexing
            i -> [w414]
            n205 = Increment(x=w414) -> (x+1=w413:i32)
            n206 = Bundle(w412, w413) -> (w411:cluster{string, i32})  [unwired: 1 in]
          }
          n207 = property on="Preset Auto" class="Ring (strict)"("StringsAndValues[]"=w408) -> ()  [unwired: 2 in, 2 out]
        }
        n208 = for {
          tunnel: w394 -> [w421] mode=indexing
          tunnel: w396 -> [w419]
          tunnel: [w418] -> w397 if=w417
          stop <- w417 stop-if-true
          n209 = Unbundle(w421) -> (w420:string, w418:i32)
          n210 = Equal?(x=w420, y=w419) -> (x = y?=w417:bool)
        }
        n211 = property on="Preset Auto" class="Ring (strict)"("Value"=w397) -> ()  [unwired: 2 in, 2 out]
      }
    }
    n212 = property on="Auto Selection" class="Arr (strict)"("Value"=w360) -> ()  [unwired: 2 in, 2 out]
    n213 = property on="Auto Pieces" class="Ring (strict)"("StringsAndValues[]"=w365) -> ()  [unwired: 2 in, 2 out]
    n214 = for {
      tunnel: w365 -> [w387]
      tunnel: w360 -> [w386] mode=indexing
      tunnel: [w385] -> w364 mode=indexing
      n215 = for {
        tunnel: w387 -> [w392] mode=indexing
        tunnel: w386 -> [w390]
        tunnel: [w391] -> w385 if=w388
        stop <- w388 stop-if-true
        n216 = Unbundle(w392) -> ("String"=w391:string, w389:u16)
        n217 = Equal?(x=w389, y=w390) -> (x = y?=w388:bool)
      }
    }
    n218 = call-poly <vilib>:"NT Write Value.vi"("String Array"=w364, "Name"="Auto Selection") -> ()  [unwired: 9 in, 1 out]
  }
  n219 = while {
    tunnel: w120 -> [w465]
    i -> [w468]
    stop <- FALSE stop-if-true
    n220 = Wait (ms)(milliseconds to wait=u32 100) -> ()  [unwired: 1 out]
    n221 = case shown="\"Record\"" "Rec Mode" {
      tunnel: w468 -> [_ _ w483]
      tunnel: [u32 2829099 ("Base Color") u32 11141120 ("Target Color") w472] -> w464
      frame "Stop", Default {
        # "Reset the color, extra updates don't cost much"
      }
      frame "Record" {
      }
      frame "Playback" {
        # "Playback"
        n222 = Quotient & Remainder(x=w483, y=u32 50 ("milliseconds to wait")) -> (x-y*floor(x/y)=w479:u32)  [unwired: 1 out]
        n223 = Divide(x=w479, y=u32 50 ("milliseconds to wait")) -> (x/y=w476:dbl)
        n224 = Multiply(x=6.283185307179586, y=w476) -> (x*y=w481:dbl)
        n225 = Sine(x=w481) -> (sin(x)=w480:dbl)
        n226 = Absolute Value(x=w480) -> (abs(x)=w473:dbl)
        n227 = call "Interpolate RGB Color.vi"("Proportion"=w473, "Target Color"=u32 30976, "Base Color"=u32 2829099) -> ("Result Color"=w472:u32)  [unwired: 8 in]
      }
    }
    n228 = property class="Pane"(reference=w465, "PaneColor"=w464) -> ()  [unwired: 1 in, 2 out]
  }
  n229 = local write "Dashboard Tab"(T3."Match" ("Dashboard Tab")) -> ()
  n230 = while {
    tunnel: u16 1741 ("timeout ms (25000)") -> [w485]
    stop <- FALSE stop-if-true
    n231 = TCP Create Listener(10:w485) -> (0:w484:errorcluster, 3:w486:refnum<k5>)  [unwired: 4 in, 1 out]
    n232 = case shown="No Error" w484 {
      selector: w484 -> [w488 _]
      tunnel: w486 -> [w489 _]
      frame No Error {
        n233 = while {
          tunnel: w489 -> [w492]
          tunnel: w488 -> [w491]
          stop <- FALSE stop-if-true
          n234 = TCP Wait On Listener(8:w491, 11:w492) -> (0:w493:errorcluster, 4:w494:refnum<k5>)  [unwired: 2 in, 3 out]
          n235 = local write "TCP"(w494) -> ()
          n236 = case shown="No Error" w493 {
            frame No Error {
            }
            frame Error {
              n237 = Wait (ms)(milliseconds to wait=u32 1000) -> ()  [unwired: 1 out]
            }
          }
        }
      }
      frame Error {
        n238 = Wait (ms)(milliseconds to wait=u32 1000) -> ()  [unwired: 1 out]
      }
    }
  }
  n239 = global write "WPI_DashboardLogging Global.vi" "Recording"(w114) -> ()
  n240 = local write "Rec Mode"(w114) -> ()
  n241 = Current VI's Path() -> (path=w13:path)
  n242 = Strip Path(path=w13) -> (stripped path=w12:path)  [unwired: 1 out]
  n243 = Build Path(base path=w12, name or relative path="FieldImage.png") -> (appended path=w10:path)
  n244 = property on="Picture 2" class="Pict"() -> ("Draw Area Size"=w9:T29)  [unwired: 2 in, 2 out]
  n245 = call <vilib>:"Read PNG File.vi"("path to PNG file"=w10) -> ("image data"=w5:T30)  [unwired: 8 in, 2 out]
  n246 = Unbundle By Name(w5) -> ("Rectangle.right"=w7:i16)
  n247 = call "Empty Picture"() -> ("empty picture"=w3:picture)
  n248 = Unbundle By Name(w9) -> ("Width"=w8:u32)
  n249 = call <vilib>:"Unflatten Pixmap.vi"("image data"=w5) -> ("24-bit pixmap"=w4:u32[][])  [unwired: 4 in, 6 out]
  n250 = Divide(x=w8, y=w7) -> (x/y=w6:dbl)
  n251 = call-poly <vilib>:"Draw Unflattened Pixmap.vi"("picture"=w3, "top left point(0, 0)"=cluster{"x":i16, "y":i16} {"x"=0, "y"=744}, "data (RGB format)"=w4) -> ("new picture"=w1:picture)  [unwired: 6 in]
  n252 = property on="Picture 2" class="Pict"("ZoomFactor"=w6) -> ()  [unwired: 2 in, 2 out]
  n253 = while {
    tunnel: w1 -> [w503]
    stop <- FALSE stop-if-true
    n254 = call-poly <vilib>:"NT Read Value.vi"("Name"="Path Data for Display") -> ("error out"=w505:errorcluster, "Variant"=w506:variant)  [unwired: 9 in]
    n255 = Variant To Data(error in=w505, type=T31 [], Variant=w506) -> (data=w504:T31)  [unwired: 1 out]
    n256 = for {
      tunnel: w504 -> [w517] mode=indexing
      shift-right: [w509] -> w498
      shift-left: w503 -> [w511]
      n257 = Unbundle(w517) -> ("Trajectory Data"=w514:T12, "Points"=w513:cluster{"x":dbl, "y":dbl, "th":dbl}[])
      n258 = control-ref of="Picture 2"() -> (w512:refnum<vi>)
      n259 = call "Draw Trajectory.vi"("new picture in"=w511, "Trajectory Data"=w514, "Picture in"=w512) -> ("Output Point"=w516:T21, "new picture"=w510:picture)  [unwired: 7 in]
      n260 = call "Draw Shapes.vi"("Output Point"=w516, "Results"=T13 {"Index"=0, "Pt Test Results"=enum."Miss"}, "new picture in"=w510, "Points"=w513, "Picture in"=w512) -> ("new picture out"=w509:picture)  [unwired: 6 in]
    }
    n261 = call <vilib>:"Picture to Pixmap.vi"("picture"=w498) -> ("image data"=w499:T30)  [unwired: 9 in, 1 out]
    n262 = call <vilib>:"Unflatten Pixmap.vi"("image data"=w499) -> ("24-bit pixmap"=w500:u32[][])  [unwired: 4 in, 6 out]
    n263 = call-poly <vilib>:"Draw Unflattened Pixmap.vi"("picture"=w498, "data (RGB format)"=w500) -> ("new picture"=→"Picture 2":picture)  [unwired: 7 in]
    n264 = Wait (ms)(milliseconds to wait=u32 1000) -> ()  [unwired: 1 out]
  }
  n265 = control-ref of="Picture 2"() -> (w20:refnum<vi>)
  n266 = property class="App"() -> ("Disp.WkSpace"=w81:T32)  [unwired: 2 in, 2 out]
  n267 = Current VI's Path() -> (path=w92:path)
  n268 = Open VI Reference(vi path=w92) -> (vi reference=w78:refnum<vi>, error out=w91:errorcluster)  [unwired: 5 in]
  n269 = Unbundle(w81) -> ("Left"=w85:i16, "Top"=w84:i16, "Right"=w62:i16, "Bottom"=w83:i16)
  n270 = Subtract(x=w83, y=i16 200) -> (x-y=w72:i16)
  n271 = Subtract(x=w72, y=i16 85) -> (x-y=w71:i16)
  n272 = Bundle(cluster=w81, "Left"=w85, "Top"=w84, "Right"=w62, "Bottom"=w72) -> (w80:T32)
  n273 = Bundle(cluster=cluster{"Width":i16, "Height":i16} {"Width"=0, "Height"=0}, "Width"=w62, "Height"=w71) -> (w47:cluster{"Width":i16, "Height":i16})
  n274 = property class="VI"(reference=w78, error in=w91, "Front Panel.WinBounds"=w80, "Front Panel.TitleBarVis"=FALSE ("Front Panel Window:Title Bar Visible"), "Front Panel.ShowMenuBar"=FALSE ("Front Panel Window:Show Menu Bar"), "Front Panel.Closeable"=FALSE ("Front Panel Window:Closeable"), "Front Panel.Resizeable"=FALSE ("Front Panel Window:Resizable"), "Front Panel.Minimizeable"=TRUE ("Front Panel Window:Minimizable"), "Front Panel.KeepWinProps"=TRUE ("Front Panel Window:Keep Window Proportions")) -> ()  [unwired: 2 out]
  n275 = property class="VI"(reference=w78) -> ("Panel"=w77:refnum<vi>)  [unwired: 1 in, 2 out]
  n276 = property class="Pnl"(reference=w77) -> ("Panes[]"=w76:refnum<vi>[])  [unwired: 1 in, 2 out]
  n277 = control-ref of="Dashboard Tab"() -> (w73:refnum<vi>)
  n278 = Index Array(array=w76, index=0) -> (element=w74:refnum<vi>)
  n279 = property class="Pane"(reference=w74, "Origin"=w67) -> ()  [unwired: 1 in, 2 out]
  n280 = property class="TabCtl (strict)"(reference=w73, "Position"=w67, "PaneDimension"=w47) -> ()  [unwired: 1 in, 2 out]
  n281 = in-place {
    in-place-border: w67 -> [w523]
    in-place-border: [w522] -> w17
    in-place-border: w66 -> [w518]
    n282 = Unbundle(w523) -> ("X"=w521:i32, "Y"=w520:i32)
    n283 = Add(x=w520, y=w518) -> (x+y=w519:i32)
    n284 = Bundle(cluster=w523, "X"=w521, "Y"=w519) -> (w522:cluster{"X":i32, "Y":i32})
  }
  n285 = in-place {
    in-place-border: w47 -> [w533]
    in-place-border: [w532] -> w19
    in-place-border: w66 -> [w529]
    n286 = Unbundle(w533) -> ("Width"=w526:i16, "Height"=w531:i16)
    n287 = Subtract(x=w531, y=w529) -> (x-y=w530:i32)
    n288 = Subtract(x=w526, y=i16 10) -> (x-y=w524:i16)
    n289 = Add(x=w530, y=15 ("x")) -> (x+y=w528:i32)
    n290 = Bundle(cluster=w533, "Width"=w524, "Height"=w528) -> (w532:cluster{"Width":i16, "Height":i16})
  }
  n291 = disable-structure shown="Disabled" {
    disable-tunnel: w20 -> [w547 _]
    disable-tunnel: w19 -> [w546 _]
    disable-tunnel: w17 -> [w536 _]
    frame Disabled {
      (unwired) FALSE
      n292 = Unbundle(w536) -> ("X"=w545:i32, "Y"=w540:i32)
      n293 = Compound Arithmetic op=ADD(20 ("value"), w540) -> (w538:i32)
      n294 = Unbundle(w546) -> ("Width"=w543:i16)  [unwired: 1 out]
      n295 = Divide(x=w543, y=i16 3) -> (x/y=w544:dbl)
      n296 = Compound Arithmetic op=ADD(w544, w545) -> (w537:dbl)
      n297 = Bundle(w537, w538) -> (w541:cluster{dbl, i32})  [unwired: 1 in]
      n298 = property class="Pict"(reference=w547, "Origin"=T33 {"Horizontal"=0, "Vertical"=750}, "Draw Area Size"=T29 {"Width"=550, "Height"=702}, "Position"=w541) -> ()  [unwired: 1 in, 2 out]
    }
    frame Enabled {
    }
  }
  n299 = control-ref of="Camera Perf"() -> (w18:refnum<vi>)
  n300 = disable-structure shown="Disabled" {
    disable-tunnel: w19 -> [w549 _]
    disable-tunnel: w17 -> [w548 _]
    frame Disabled {
      n301 = control-ref of="Drive Base"() -> (w556:refnum<vi>)
      n302 = Unbundle(w549) -> ("Width"=w552:i16)  [unwired: 1 out]
      n303 = Unbundle(w548) -> ("X"=w554:i32)  [unwired: 1 out]
      n304 = Divide(x=w552, y=i16 2) -> (x/y=w551:dbl)
      n305 = Build Array(w556) -> (w550:refnum<vi>[], w561:refnum<vi>, w560:refnum<vi>, w559:refnum<vi>, w558:refnum<vi>, w557:refnum<vi>)
      n306 = Compound Arithmetic op=ADD(w551, w554) -> (w555:dbl)
      n307 = for {
        tunnel: w550 -> [w564] mode=indexing
        tunnel: w555 -> [w572]
        i -> [w568]
        n308 = Multiply(x=w568, y=50.0) -> (x*y=w569:dbl)
        n309 = Add(x=w569, y=100.0) -> (x+y=w567:dbl)
        n310 = Bundle(cluster=cluster{"X":i32, "Y":i32} {"X"=0, "Y"=0}, "X"=w572, "Y"=w567) -> (w566:cluster{"X":i32, "Y":i32})
        n311 = property class="Bool (strict)"(reference=w564, "Position"=w566, "Button Size"=cluster{"Width":u32, "Height":u32} {"Width"=30, "Height"=30}, "DisabledEnum"=T34."Disabled" ("Disabled")) -> ()  [unwired: 1 in, 2 out]
      }
    }
    frame Enabled {
    }
  }
  n312 = in-place {
    in-place-border: w19 -> [w579]
    in-place-border: [w578] -> _
    w575 = 2.5 ("y")
    n313 = Unbundle(w579) -> ("Width"=w577:i16, "Height"=w576:i16)
    n314 = Divide(x=w576, y=w575) -> (x/y=w573:dbl)
    n315 = Divide(x=w577, y=w575) -> (x/y=w574:dbl)
    n316 = Bundle(cluster=w579, "Width"=w574, "Height"=w573) -> (w578:cluster{"Width":i16, "Height":i16})
  }
  n317 = control-ref of="Endgame?"() -> (w69:refnum<vi>)
  n318 = Unbundle(w17) -> ("X"=w21:i32)  [unwired: 1 out]
  n319 = Unbundle(w19) -> ("Width"=w49:i16, "Height"=w53:i16)
  n320 = Unbundle(w17) -> ("X"=w35:i32, "Y"=w32:i32)
  n321 = Unbundle(w47) -> ("Height"=w46:i16)  [unwired: 1 out]
  n322 = Unbundle(w19) -> ("Width"=w27:i16, "Height"=w24:i16)
  n323 = Divide(x=w49, y=i16 2) -> (x/y=w60:dbl)
  n324 = Compound Arithmetic op=unknown(10 ("value"), w35) -> (w33:i32)
  n325 = property class="Bool (strict)"(reference=w69, "Position"=w17, "Button Size"=w19) -> ()  [unwired: 1 in, 2 out]
  n326 = Add(x=w46, y=i16 40) -> (x+y=w15:i16)
  n327 = Divide(x=w49, y=i16 3) -> (x/y=w50:dbl)
  n328 = Divide(x=w53, y=i16 3) -> (x/y=w52:dbl)
  n329 = Compound Arithmetic op=unknown(50 ("value"), w32) -> (w30:i32)
  n330 = Divide(x=w27, y=i16 2) -> (x/y=w25:dbl)
  n331 = Compound Arithmetic op=ADD(w21, 200.0 ("value"), w60) -> (w58:dbl)
  n332 = disable-structure shown="Disabled" {
    disable-tunnel: [w583 _] -> w63
    disable-tunnel: w19 -> [w581 _]
    disable-tunnel: w17 -> [w580 _]
    frame Disabled {
      w587 = i16 10 ("y")
      n333 = in-place {
        in-place-border: w581 -> [w611]
        in-place-border: [w610] -> w582
        in-place-border: w587 -> [w608]
        in-place-border: 1.5 ("y") -> [w605]
        in-place-border: [w603] -> w585
        in-place-border: [w602] -> w584
        n334 = Unbundle(w611) -> ("Width"=w602:i16, "Height"=w609:i16)
        n335 = Multiply(x=w608, y=i16 2) -> (x*y=w607:i16)
        n336 = Subtract(x=w609, y=w607) -> (x-y=w604:i16)
        n337 = Multiply(x=w605, y=w604) -> (x*y=w603:dbl)
        n338 = Bundle(cluster=w611, "Width"=w603, "Height"=w604) -> (w610:cluster{"Width":i16, "Height":i16})
      }
      n339 = in-place {
        in-place-border: w580 -> [w601]
        in-place-border: [w600] -> w583
        in-place-border: w587 -> [w597]
        in-place-border: w585 -> [w596]
        in-place-border: w584 -> [w590]
        n340 = Unbundle(w601) -> ("X"=w594:i32, "Y"=w599:i32)
        n341 = Divide(x=w596, y=2.0) -> (x/y=w595:dbl)
        n342 = Divide(x=w590, y=2.0) -> (x/y=w589:dbl)
        n343 = Add(x=w599, y=w597) -> (x+y=w598:i32)
        n344 = Compound Arithmetic op=ADD(w594, invert w595, w589) -> (w593:dbl)
        n345 = Bundle(cluster=w601, "X"=w593, "Y"=w598) -> (w600:cluster{"X":i32, "Y":i32})
      }
      n346 = control-ref of="Camera Image Right"() -> (w588:refnum<vi>)
      n347 = property class="ImageControl"(reference=w588, "Position"=w583, "Image Area Size"=w582) -> ()  [unwired: 1 in, 2 out]
    }
    frame Enabled {
    }
  }
  n348 = Bundle(cluster=w19, "Width"=w25, "Height"=w24) -> (w23:cluster{"Width":i16, "Height":i16})
  n349 = Bundle(cluster=w17, "X"=w33, "Y"=w30) -> (w29:cluster{"X":i32, "Y":i32})
  n350 = Bundle(cluster=w17, "X"=w33, "Y"=w32) -> (w36:cluster{"X":i32, "Y":i32})
  n351 = Bundle(cluster=w17, "X"=i16 400 ("y"), "Y"=w15) -> (w38:cluster{"X":i32, "Y":i32})
  n352 = Bundle(cluster=w17, "X"=i16 230 ("y"), "Y"=w15) -> (w40:cluster{"X":i32, "Y":i32})
  n353 = Bundle(cluster=w17, "X"=0, "Y"=w15) -> (w44:cluster{"X":i32, "Y":i32})
  n354 = Bundle(cluster=w17, "X"=w58, "Y"=100.0) -> (w56:cluster{"X":i32, "Y":i32})
  n355 = Bundle(cluster=w19, "Width"=w50, "Height"=w52) -> (w55:cluster{"Width":i16, "Height":i16})
  n356 = Bundle(cluster=w17, "X"=600, "Y"=w15) -> (w16:cluster{"X":i32, "Y":i32})
  n357 = disable-structure shown="Disabled" {
    disable-tunnel: w36 -> [w613 _]
    disable-tunnel: w29 -> [w612 _]
    frame Disabled {
      n358 = control-ref of="IMU Angle"() -> (w615:refnum<vi>)
      n359 = property class="DigNum (strict)"(reference=w615, "Position"=w612) -> ()  [unwired: 1 in, 2 out]
      n360 = property class="Enum (strict)"("Position"=w613) -> (reference=w614:refnum<vi>)  [unwired: 1 in, 2 out]
    }
    frame Enabled {
    }
  }
  n361 = control-ref of="Tree"() -> (w28:refnum<vi>)
  n362 = control-ref of="Rec Mode"() -> (w37:refnum<vi>)
  n363 = control-ref of="DB Camera Config"() -> (w41:refnum<vi>)
  n364 = control-ref of="Camera Name Right"() -> (w48:refnum<vi>)
  n365 = disable-structure shown="Disabled" {
    disable-tunnel: w56 -> [w617 _]
    disable-tunnel: w55 -> [w616 _]
    frame Disabled {
      n366 = control-ref of="Errors"() -> (w618:refnum<vi>)
      n367 = property class="Str"(reference=w618, "Position"=w617, "Size"=w616) -> ()  [unwired: 1 in, 2 out]
    }
    frame Enabled {
    }
  }
  n368 = property class="RadioBtnsControl (strict)"(reference=w37, "Position"=w38) -> ()  [unwired: 1 in, 2 out]
  n369 = property class="Str"(reference=w18, "Position"=w16) -> ()  [unwired: 1 in, 2 out]
  n370 = property class="Bool (strict)"(reference=w41, "Position"=w40) -> ()  [unwired: 1 in, 2 out]
  n371 = property class="Tree (strict)"(reference=w28, "Position"=cluster{"Left":i32, "Top":i32} {"Left"=10, "Top"=35}, "Size"=w23) -> ()  [unwired: 1 in, 2 out]
  n372 = control-ref of="Time Remaining"() -> (w65:refnum<vi>)
  n373 = property class="CmbBox"(reference=w48, "Position"=w44) -> ()  [unwired: 1 in, 2 out]
  n374 = property class="DigNum (strict)"(reference=w65) -> ("Bounds"=w64:T29)  [unwired: 1 in, 2 out]
  n375 = disable-structure shown="Disabled" {
    disable-tunnel: w65 -> [w623 _]
    disable-tunnel: w64 -> [w622 _]
    disable-tunnel: w63 -> [w621 _]
    disable-tunnel: w19 -> [w620 _]
    disable-tunnel: w17 -> [w619 _]
    frame Disabled {
      n376 = in-place {
        in-place-border: w619 -> [w647]
        in-place-border: [w646] -> w624
        in-place-border: w620 -> [w643]
        in-place-border: w622 -> [w639]
        in-place-border: w621 -> [w635]
        n377 = Unbundle(w647) -> ("X"=w626:i32, "Y"=w644:i32)
        n378 = Unbundle(w643) -> ("Height"=w641:i16)  [unwired: 1 out]
        n379 = Unbundle(w635) -> ("X"=w632:i32)  [unwired: 1 out]
        n380 = Unbundle(w639) -> ("Width"=w633:u32, "Height"=w637:u32)
        n381 = Divide(x=w641, y=2.0) -> (x/y=w640:dbl)
        n382 = Compound Arithmetic op=ADD(invert w626, w632) -> (w630:i32)
        n383 = Divide(x=w637, y=2.0) -> (x/y=w636:dbl)
        n384 = Divide(x=w633, y=2.0) -> (x/y=w628:dbl)
        n385 = Divide(x=w630, y=2.0) -> (x/y=w629:dbl)
        n386 = Subtract(x=w629, y=w628) -> (x-y=w627:dbl)
        n387 = Add(x=w626, y=w627) -> (x+y=w625:dbl)
        n388 = Compound Arithmetic op=ADD(w644, invert w636, w640) -> (w645:dbl)
        n389 = Bundle(cluster=w647, "X"=w625, "Y"=w645) -> (w646:cluster{"X":i32, "Y":i32})
      }
      n390 = property class="DigNum (strict)"(reference=w623, "Position"=w624) -> ()  [unwired: 1 in, 2 out]
    }
    frame Enabled {
    }
  }
